vi "Pre Launch Init.vi"(11 "Cooler UI with Events in":refnum<class "Cooler UI with Events.lvclass"> caption="Acteur en entrée") -> (0 "error out":errorcluster caption="sortie d'erreur", 3 "Cooler UI with Events out":refnum<class "Cooler UI with Events.lvclass"> caption="Acteur en sortie")   [LabVIEW 2015, in "Cooler UI.lvlib" / "Cooler UI with Events.lvclass"]
doc: "(<B>Nom de fichier</B> : Actor Framework.lvlib:Actor.lvclass:Pre Launch Init.vi)\n\nDéfinit le comportement entre le moment où la méthode Lancer un acteur imbriqué est appelée et le moment qui précède l'exécution de la méthode Noyau d'acteur.\n\nPar défaut, cette méthode ne fait rien. Une classe descendante peut la redéfinir pour configurer un comportement."
uses:
  Cooler UI with Events.lvclass
  Status.ctl
  Cooler UI with Events.lvclass/Cooler UI with Events.ctl
  <vilib>/ActorFramework/Actor/Actor.lvclass
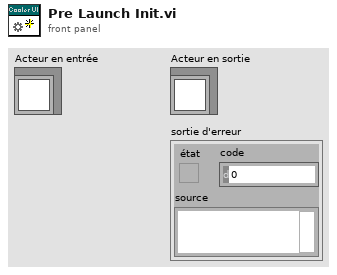
[diagram p1: front panel]
types:
  T1 = typedef "Cooler UI.lvlib/Cooler UI with Events.lvclass/Status.ctl" = cluster{"Fan A":cluster{"State":bool, "Fault":bool}, "Fan B":cluster{"State":bool, "Fault":bool}}
  T2 = cluster{"Fan Status":refnum<user-event>, "Temperature":refnum<user-event>, "Pump":refnum<user-event>}
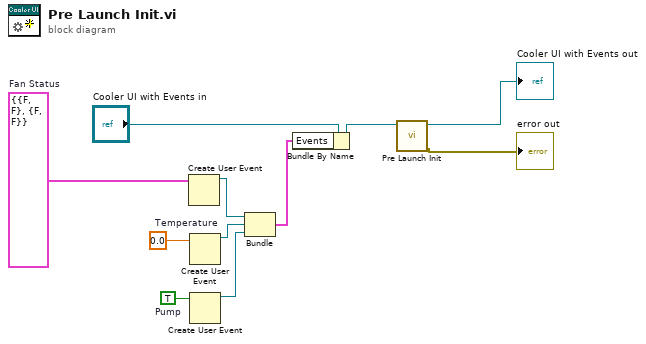
[diagram p0: block diagram]
diagram:
  w5 = T1 {"Fan A"={"State"=FALSE, "Fault"=FALSE}, "Fan B"={"State"=FALSE, "Fault"=FALSE}}  # Fan Status
  w6 = 0.0  # Temperature
  w7 = TRUE  # Pump
  n1 = Create User Event(user event datatype=w5) -> (user event=w3:refnum<user-event>)  [unwired: 1 in, 1 out]
  n2 = Create User Event(user event datatype=w6) -> (user event=w4:refnum<user-event>)  [unwired: 1 in, 1 out]
  n3 = Create User Event(user event datatype=w7) -> (user event=w2:refnum<user-event>)  [unwired: 1 in, 1 out]
  n4 = Bundle("Fan Status"=w3, "Temperature"=w4, "Pump"=w2) -> (w1:T2)  [unwired: 1 in]
  n5 = Bundle By Name(cluster="Cooler UI with Events in", "Events"=w1) -> (w8:refnum<class "Cooler UI with Events.lvclass">)
  n6 = call-parent "Pre Launch Init.vi"("Actor in"=w8) -> ("error out"=→"error out":errorcluster, "Actor out"=→"Cooler UI with Events out":refnum<class "Cooler UI with Events.lvclass">)  [unwired: 9 in]
